vi "Frame1.vi"   [LabVIEW 2014]
uses:
  QwaveSys_Interface/QwaveSys_Interface.lvlib
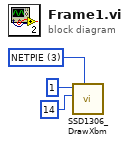
[diagram p0: block diagram]
diagram:
  w1 = u16 3 items=["WiFi Logo", "Active Symbole", "Inactive Symbole", "NETPIE"] ("xbm")
  n1 = call "SSD1306_DrawXbm.vi"("xbm"=w1, "y"=u8 14, "x"=u8 1) -> ()  [unwired: 8 in, 1 out]
